vi "Elevator - State Process.vi"(8 "error in (no error)":errorcluster, 11 "View Model":T1) -> (0 "error out":errorcluster, 3 "View Model":T1)   [LabVIEW 2017]
doc: "Perform actions specific to a state"
uses:
  View Model/Controls/View Model.ctl
  Configuration/Controls/Config Model.ctl
  Configuration/Controls/Config Data.ctl
  Error Handler/Controls/Error Model.ctl
  Error Handler/Controls/Error Data.ctl
  Error Handler/Controls/Error Type.ctl
  View Model/Controls/Shared Model.ctl
  Controls/Elevator Model.ctl
  Controls/Elevator Location.ctl
  Controls/Elevator CMD Data.ctl
  Controls/Elevator Commands.ctl
  Controls/Elevator Overhead.ctl
  Controls/Elevator States.ctl
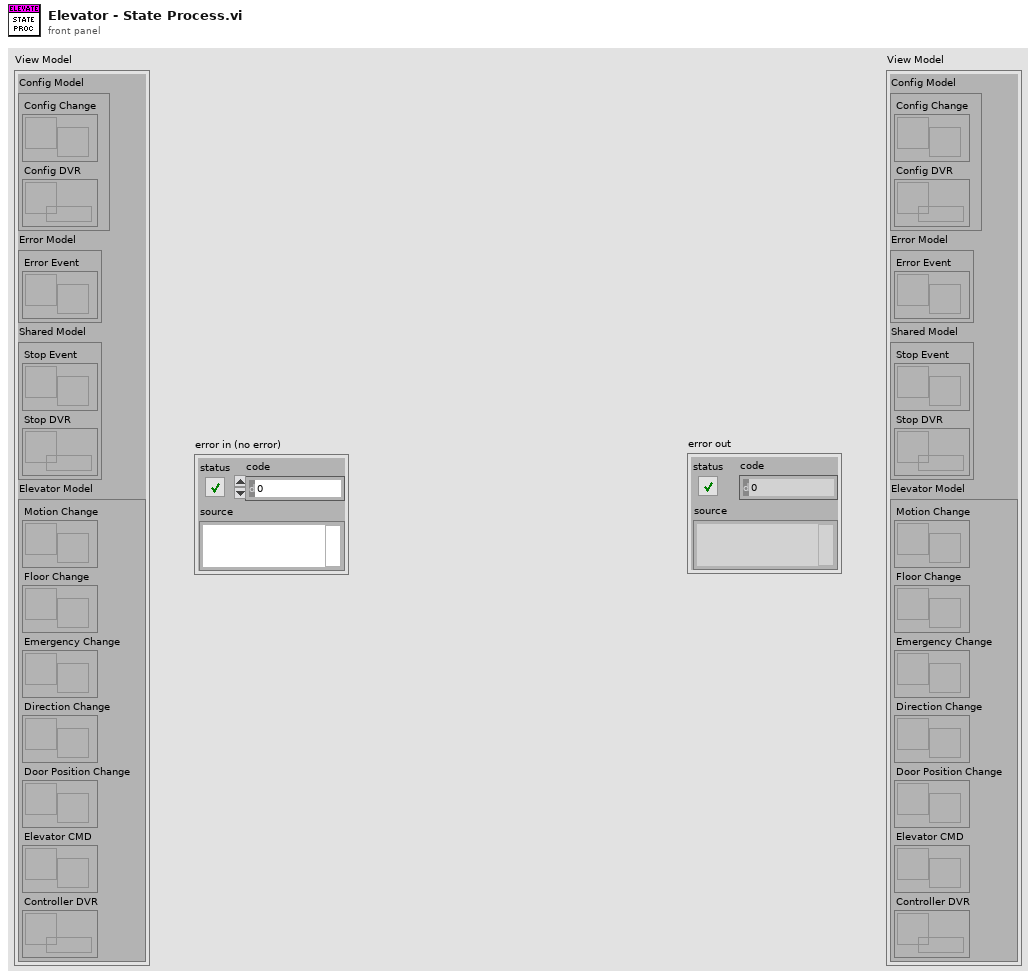
[diagram p1: front panel]
types:
  T1 = typedef "View Model.ctl" = cluster{"Config Model":T2, "Error Model":T3, "Shared Model":T4, "Elevator Model":T5}
  T2 = typedef "Config Model.ctl" = cluster{"Config Change":refnum<user-event>, "Config DVR":refnum<data-value>}
  T3 = typedef "Error Model.ctl" = cluster{"Error Event":refnum<user-event>}
  T4 = typedef "Shared Model.ctl" = cluster{"Stop Event":refnum<user-event>, "Stop DVR":refnum<data-value>}
  T5 = typedef "Elevator Model.ctl" = cluster{"Motion Change":refnum<user-event>, "Floor Change":refnum<user-event>, "Emergency Change":refnum<user-event>, "Direction Change":refnum<user-event>, "Door Position Change":refnum<user-event>, "Elevator CMD":refnum<user-event>, "Controller DVR":refnum<data-value>}
  T6 = typedef "Elevator States.ctl" = enum16{"Initial", "Wait for 1st Request", "Start and Move", "Analysis", "Continue Travel", "Stop at Floor", "Open and Close Door", "No Request", "Emergency", "Terminate"}
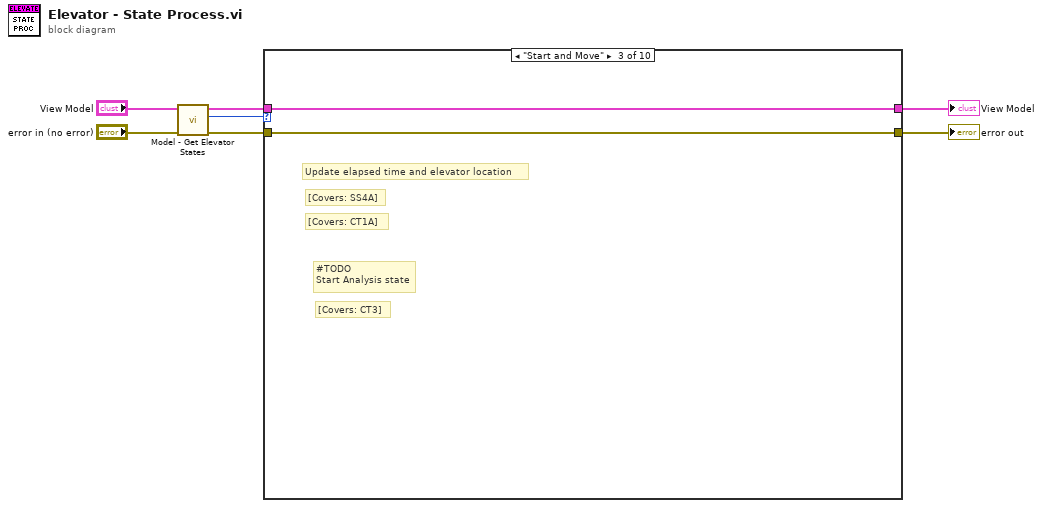
[diagram p0: block diagram]
diagram:
  n1 = call "Model - Get Elevator States.vi"("error in (no error)"="error in (no error)", "View Model"="View Model") -> ("error out"=w3:errorcluster, "Elevator State"=w5:T6, "View Model"=w4:T1)  [unwired: 6 in, 1 out]
  n2 = case shown="\"Start and Move\"" w5 {
    tunnel: w4 -> [w9 w11 w13 w15 w17 w19 w21 w23 w25 w27]
    tunnel: w3 -> [w8 w10 w12 w14 w16 w18 w20 w22 w24 w26]
    tunnel: [w9 w11 w13 w15 w17 w19 w21 w23 w25 w27] -> w2
    tunnel: [w8 w10 w12 w14 w16 w18 w20 w22 w24 w26] -> w1
    frame "Initial", Default {
      # "[Covers: NR1]"
      # "Countdown inactivity timer to zero if >0."
      # "[Covers: WS1]"
      # "Maintain initial state defaults"
    }
    frame "Wait for 1st Request" {
    }
    frame "Start and Move" {
      # "[Covers: CT3]"
      # "#TODO\nStart Analysis state"
      # "[Covers: CT1A]"
      # "[Covers: SS4A]"
      # "Update elapsed time and elevator location"
    }
    frame "Analysis" {
    }
    frame "Continue Travel" {
    }
    frame "Stop at Floor" {
    }
    frame "Open and Close Door" {
      # "[Covers: SS1]"
      # "Send digital output to open doors. Fire door open event"
    }
    frame "No Request" {
    }
    frame "Emergency" {
    }
    frame "Terminate" {
    }
  }
  "View Model" <- w2
  "error out" <- w1
